vi "Cleanup Session.vi"(8 "error in":errorcluster, 11 "Plugin in":refnum<class "Performanced XNET CAN Signal Logger.lvclass">) -> (0 "error out":errorcluster, 3 "Plugin out":refnum<class "Performanced XNET CAN Signal Logger.lvclass">)   [LabVIEW 2021, in "Performanced XNET CAN Signal Logger.lvlib" / "Performanced XNET CAN Signal Logger.lvclass"]
uses:
  Performanced XNET CAN Signal Logger.lvclass
  <userlib>/_NEVSTOP/GlobalStop/_gStop.vi
  Performanced XNET CAN Signal Logger.lvclass/Performanced XNET CAN Signal Logger.ctl
  <userlib>/_NEVSTOP/GlobalStop/GSTOP.lvlib
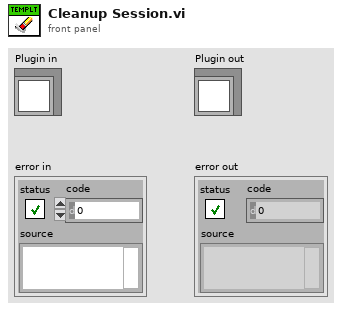
[diagram p1: front panel]
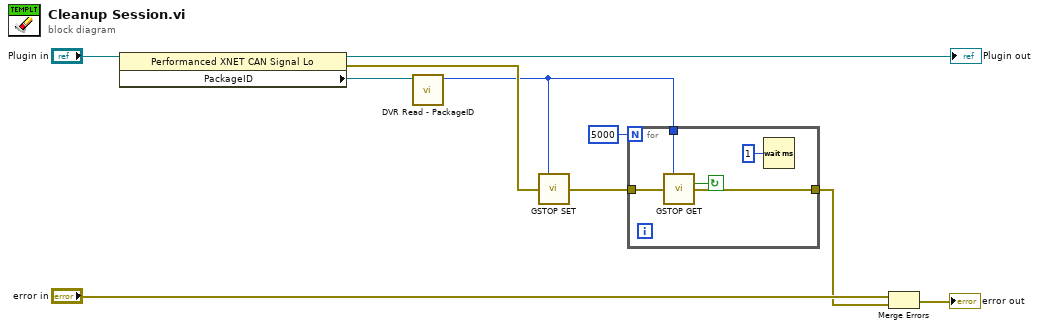
[diagram p0: block diagram]
diagram:
  n1 = property class="Performanced XNET CAN Signal Lo"(reference="Plugin in") -> (reference out=→"Plugin out":refnum<class "Performanced XNET CAN Signal Logger.lvclass">, error out=w6:errorcluster, "PackageID"=w3:refnum<data-value>)  [unwired: 1 in]
  n2 = call "DVR Read - PackageID.vi"("Data Value Reference in"=w3) -> ("PackageID"=w1:i32)  [unwired: 10 in]
  n3 = call <userlib>:"GSTOP SET.vi"("index(-1 for All)"=w1, "error in (no error)"=w6) -> ("error out"=w5:errorcluster)  [unwired: 13 in]
  n4 = for {
    N: 5000 -> [_]
    tunnel: w5 -> [w15]
    tunnel: [w14] -> w4
    tunnel: w1 -> [w13]
    stop <- w11 continue-if-true
    n5 = call <userlib>:"GSTOP GET.vi"("index(-1 for All)"=w13, "error in (no error)"=w15) -> ("stop"=w11:bool, "error out"=w14:errorcluster)  [unwired: 12 in]
    n6 = Wait (ms)(milliseconds to wait=u32 1) -> ()  [unwired: 1 out]
  }
  n7 = Merge Errors("error in", w4) -> (→"error out":errorcluster)
